vi "ExtendedKalmanFilter_Correct.vi"(4 "H_FuncExtra":variant, 6 "H_Func":T1, 7 "Rows":i32, 8 "R":T2, 9 "Y":T2, 10 "U":T2, 11 "in ExtendedKalmanFiilter":T3) -> (0 "Error":bool, 3 "out ExtendedKalmanFiilter":T3)   [LabVIEW 2019, in "Trajectory_Library.lvlib"]
doc: "Correct the state estimate x-hat using the measurements in y.\n \nThis is useful for when the measurements available during a timestep's Correct() call vary. \n\nInputs:\n - inExtendedKalmanFIlter -- filter data cluster\n - rows -- Number of rows in the result of f(x, u).\n - u -- Same control input used in the predict step.\n - y -- Measurement vector.\n - R -- Discrete measurement noise covariance matrix.\n - h_Func -- A vector-valued function reference of x and u that returns the measurement vector.\n - H_func_extra -- extra data, if any, used by H_Func\n\nReturns:\n - outExtendedKalmanFIlter -- updated filter data cluster\n - error -- If TRUE, an error occured."
uses:
  Trajectory_Library.lvlib
  TypeDef/EXTENDED_KALMAN_FILTER.ctl
  <vilib>/Analysis/Matrix/Datatypes/RealMatrix.ctl
  TypeDef/CALLBACK_FUNC_TYPE.ctl
  <vilib>/Analysis/7linalg.llb/Real Transpose Matrix.vi
  <vilib>/Analysis/baseanly.llb/Real A x B.vi
  MatBuilder_Create.vi
  <vilib>/Analysis/7linalg.llb/Create Special Matrix.vi
  <vilib>/Analysis/7linalg.llb/Create Special Real Matrix.vi
  <vilib>/Analysis/Matrix/Numeric/Subtract/Subtract - RM,RM.vi
  <vilib>/Analysis/Matrix/Numeric/Add/Add - RM,RM.vi
  <vilib>/Analysis/7linalg.llb/Solve Linear Equations (multiple right hand).vi
  <vilib>/Analysis/Matrix/NI_Matrix.lvlib
  <vilib>/Analysis/NI_AALPro.lvlib
  <vilib>/Analysis/NI_AALBase.lvlib
panel:
  # "<Inputs, 1>"
  # "<Rows, 1>"
  # "<Rows, Rows>"
  # "State Estimate <Statess,1>"
  # "<States, States>"
  # "<States, States>"
  # "<Statess,  States>"
  # "<Outputs, Outputs>"
  # "State Estimate <Statess,1>"
  # "<States, States>"
  # "<States, States>"
  # "<Statess,  States>"
  # "<Outputs, Outputs>"
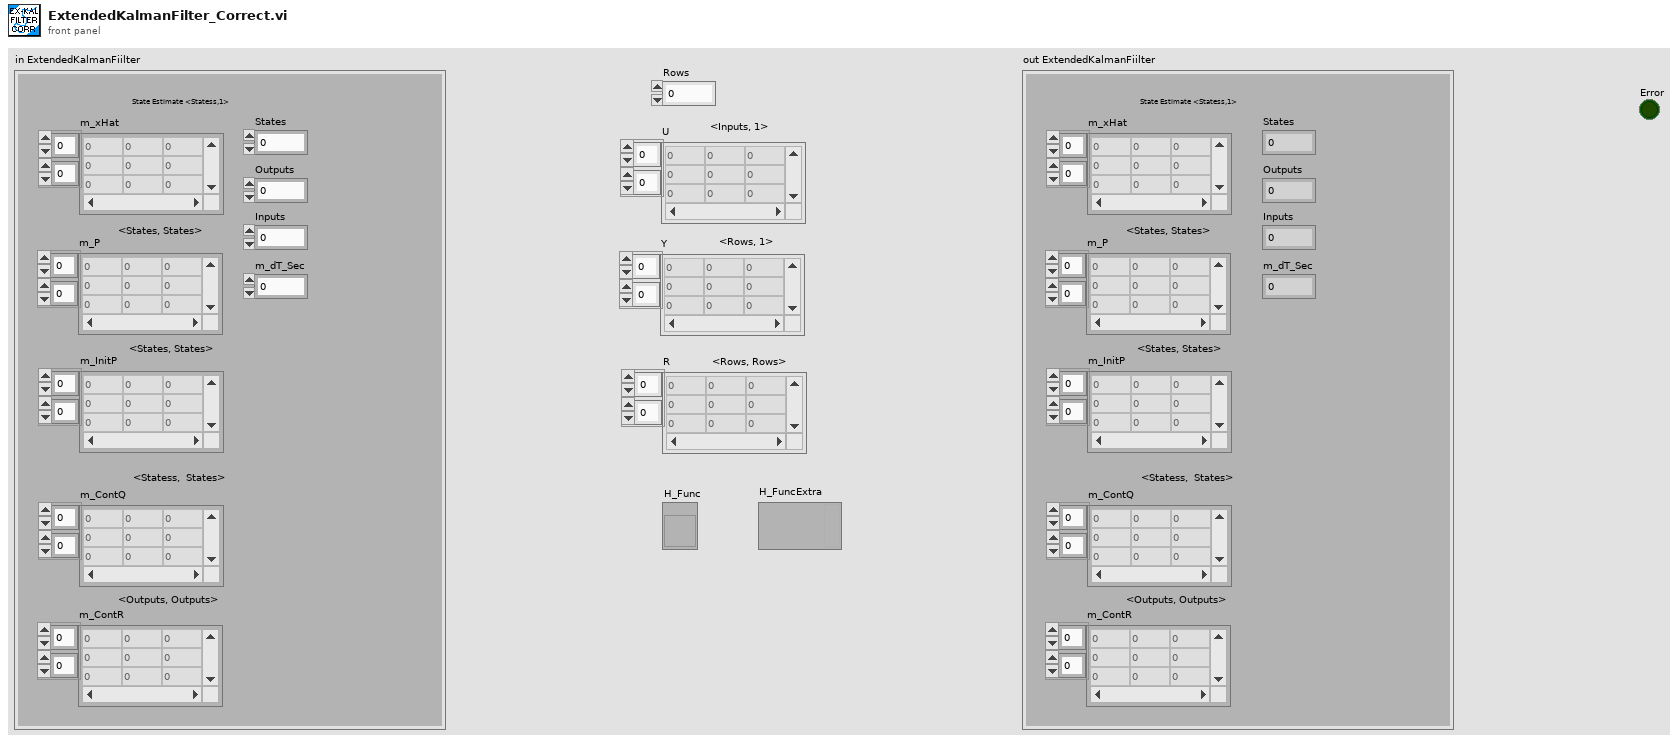
[diagram p1: front panel]
types:
  T1 = typedef "Trajectory_Library.lvlib/CALLBACK_FUNC_TYPE.ctl" = refnum<vi>
  T2 = typedef "NI_Matrix.lvlib/RealMatrix.ctl" = dbl[][]
  T3 = typedef "Trajectory_Library.lvlib/EXTENDED_KALMAN_FILTER.ctl" = cluster{"m_P":T2, "m_xHat":T2, "States":i32, "Outputs":i32, "m_ContR":T2, "m_ContQ":T2, "m_dT_Sec":dbl, "Inputs":i32, "m_InitP":T2}
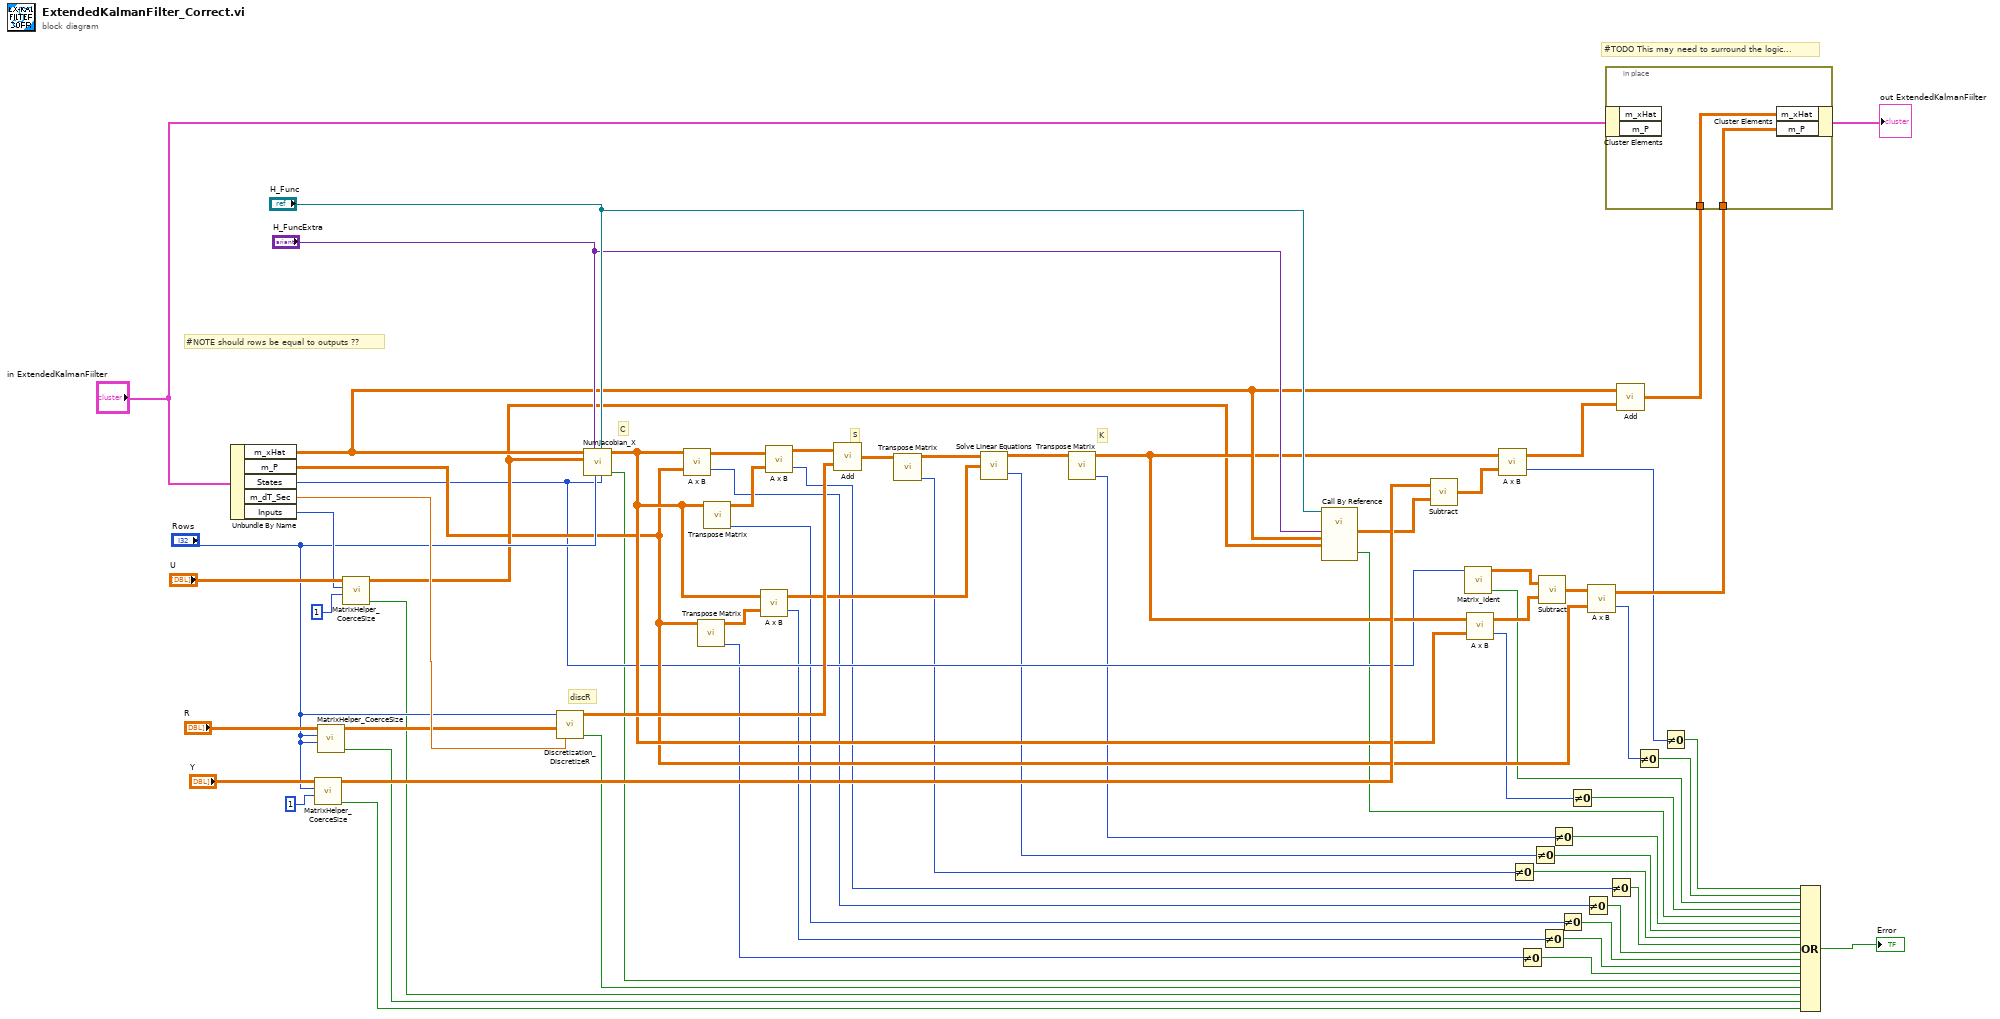
[diagram p0: block diagram]
diagram:
  # "K"
  # "S"
  # "C"
  # "#NOTE should rows be equal to outputs ??"
  # "#TODO This may need to surround the logic..."
  # "discR"
  n1 = Unbundle By Name("in ExtendedKalmanFiilter") -> ("m_xHat"=w39:T2, "m_P"=w29:T2, "States"=w28:i32, "m_dT_Sec"=w65:dbl, "Inputs"=w58:i32)
  n2 = call "MatrixHelper_CoerceSize.vi"("Columns"=1, "Rows"="Rows", "input matrix"="Y") -> ("Coerced"=w2:bool, "output matrix"=w41:T2)  [unwired: 7 in]
  n3 = call "MatrixHelper_CoerceSize.vi"("Columns"="Rows", "Rows"="Rows", "input matrix"="R") -> ("Coerced"=w4:bool, "output matrix"=w54:T2)  [unwired: 7 in]
  n4 = call "MatrixHelper_CoerceSize.vi"("Columns"=1, "Rows"=w58, "input matrix"="U") -> ("Coerced"=w3:bool, "output matrix"=w30:T2)  [unwired: 7 in]
  n5 = call "Discretization_DiscretizeR.vi"("dT_Seconds"=w65, "ContR"=w54, "Outputs"="Rows") -> ("Size Coerced"=w1:bool, "DiscR"=w46:T2)  [unwired: 7 in]
  n6 = call "NumJacobian_X.vi"("States"=w28, "F_FUNC"="H_Func", "Rows"="Rows", "ExtraPassedData"="H_FuncExtra", "U"=w30, "X"=w39) -> ("Error"=w26:bool, "Result"=w34:T2)  [unwired: 4 in]
  n7 = call-poly <vilib>:"A x B.vi"("B"=w29, "A"=w34) -> ("error"=w21:i32, "A x B"=w49:T2)
  n8 = call-poly <vilib>:"Transpose Matrix.vi"("Input Matrix"=w29) -> ("error"=w25:i32, "Matrix Transpose"=w52:T2)  [unwired: 9 in]
  n9 = call-poly <vilib>:"Transpose Matrix.vi"("Input Matrix"=w34) -> ("error"=w23:i32, "Matrix Transpose"=w48:T2)  [unwired: 9 in]
  n10 = call-poly <vilib>:"A x B.vi"("B"=w52, "A"=w34) -> ("error"=w24:i32, "A x B"=w43:T2)
  n11 = call-poly <vilib>:"A x B.vi"("B"=w48, "A"=w49) -> ("error"=w20:i32, "A x B"=w47:T2)
  n12 = call-poly <vilib>:"Add.vi"("Real Matrix B"=w46, "Real Matrix A"=w47) -> ("A + B"=w45:T2)
  n13 = call-poly <vilib>:"Transpose Matrix.vi"("Input Matrix"=w45) -> ("error"=w19:i32, "Matrix Transpose"=w44:T2)  [unwired: 9 in]
  n14 = call-poly <vilib>:"Solve Linear Equations.vi"("Known Matrix"=w43, "Input Matrix"=w44) -> ("error"=w18:i32, "Solution Matrix"=w42:T2)  [unwired: 1 in]
  n15 = call-poly <vilib>:"Transpose Matrix.vi"("Input Matrix"=w42) -> ("error"=w17:i32, "Matrix Transpose"=w35:T2)  [unwired: 9 in]
  n16 = call-by-ref "?"(reference="H_Func", "U"=w30, "X"=w39, "Variant"="H_FuncExtra") -> ("Error"=w12:bool, "NewX"=w40:T2)  [unwired: 8 in, 2 out]
  n17 = call-poly <vilib>:"Subtract.vi"("Real Matrix B"=w40, "Real Matrix A"=w41) -> ("A - B"=w36:T2)
  n18 = call "Matrix_Ident.vi"("Size"=w28) -> ("Error"=w9:bool, "output matrix"=w33:T2)  [unwired: 9 in]
  n19 = call-poly <vilib>:"A x B.vi"("B"=w34, "A"=w35) -> ("error"=w11:i32, "A x B"=w32:T2)
  n20 = call-poly <vilib>:"A x B.vi"("B"=w36, "A"=w35) -> ("error"=w6:i32, "A x B"=w38:T2)
  n21 = Not Equal To 0?(x=w19) -> (x != 0?=w15:bool)
  n22 = Not Equal To 0?(x=w25) -> (x != 0?=w64:bool)
  n23 = Not Equal To 0?(x=w18) -> (x != 0?=w14:bool)
  n24 = call-poly <vilib>:"Subtract.vi"("Real Matrix B"=w32, "Real Matrix A"=w33) -> ("A - B"=w31:T2)
  n25 = Not Equal To 0?(x=w24) -> (x != 0?=w63:bool)
  n26 = Not Equal To 0?(x=w17) -> (x != 0?=w13:bool)
  n27 = Not Equal To 0?(x=w23) -> (x != 0?=w62:bool)
  n28 = Not Equal To 0?(x=w11) -> (x != 0?=w10:bool)
  n29 = Not Equal To 0?(x=w21) -> (x != 0?=w22:bool)
  n30 = call-poly <vilib>:"A x B.vi"("B"=w29, "A"=w31) -> ("error"=w8:i32, "A x B"=w27:T2)
  n31 = Not Equal To 0?(x=w20) -> (x != 0?=w16:bool)
  n32 = call-poly <vilib>:"Add.vi"("Real Matrix B"=w38, "Real Matrix A"=w39) -> ("A + B"=w37:T2)
  n33 = in-place {
    in-place-border: w27 -> [w69]
    in-place-border: w37 -> [w68]
    n34 = in-place-cluster #1("in ExtendedKalmanFiilter") -> ()  [unwired: 2 out]
    n35 = in-place-cluster #1("m_xHat"=w68, "m_P"=w69) -> (→"out ExtendedKalmanFiilter":T3)
  }
  n36 = Not Equal To 0?(x=w8) -> (x != 0?=w7:bool)
  n37 = Not Equal To 0?(x=w6) -> (x != 0?=w5:bool)
  n38 = Compound Arithmetic op=OR(w5, w7, w9, w10, w12, w13, w14, w15, w16, w22, w62, w63, w64, w26, w1, w3, w4, w2) -> (→"Error":bool)
